vi "FRCts20_Backend_SNS_Subscribe.vi"(6 "Message Attributes":T1, 8 "error in (no error)":errorcluster, 10 "Data":string, 11 "Engine_Refnums":T2) -> (0 "error out":errorcluster)   [LabVIEW 2013, in "FRCts20_Backend_Engine.lvlib"]
uses:
  FRCts20_Backend_Engine.lvlib
  FRCts20_Backend_EngineRefnums.ctl
  INI_Accessor/FRCts20_Backend_INI Controller.lvclass
  Dependencies/AMC/_SubVIs/TypeDefs/Message Queue.ctl
  Dependencies/AMC/_SubVIs/TypeDefs/Message.ctl
  Dependencies/Keyed Array/KeyedArray.ctl
  <vilib>/addons/database/Connection.llb/Conn ObjectReference.ctl
  FRCts20_Backend_FGVOperation.ctl
  FRCts20_Backend_API/FRCts20_Backend_API_SNS.ctl
  <vilib>/National Instruments/NI Amazon Web Services (AWS) Toolkit for LabVIEW/S3/vi source/Typedefs/AMZ_S3_AWS Credentials.ctl
  <vilib>/National Instruments/NI Amazon Web Services (AWS) Toolkit for LabVIEW/SNS/VI Source/AWS SNS Class/AWS_SNS.lvclass
  <vilib>/National Instruments/NI Amazon Web Services (AWS) Toolkit for LabVIEW/SNS/VI Source/Public Typedefs/AWS_SNS Subcribe Parameters.ctl
  <vilib>/National Instruments/NI Amazon Web Services (AWS) Toolkit for LabVIEW/S3/vi source/LV Interface for Amazon S3.lvlib
  <vilib>/National Instruments/NI Amazon Web Services (AWS) Toolkit for LabVIEW/SNS/VI Source/AWS_SNS.lvlib
  FRCts20_Backend_API/FRCts20_Backend_API.lvlib
  Dependencies/Keyed Array/Tools_KeyedArray.lvlib
  Dependencies/AMC/AMC.lvlib
  <vilib>/addons/database/NI_Database_API.lvlib
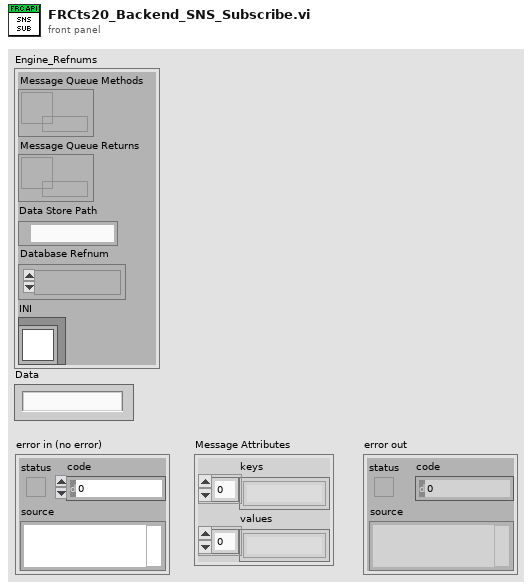
[diagram p1: front panel]
types:
  T1 = typedef "Tools_KeyedArray.lvlib/KeyedArray.ctl" = cluster{"keys":string[], "values":string[]}
  T2 = typedef "FRCts20_Backend_Engine.lvlib/FRCts20_Backend_EngineRefnums.ctl" = cluster{"Message Queue Methods":T3, "Message Queue Returns":T3, "Data Store Path":path, "Database Refnum":T4, "INI":refnum<class "FRCts20_Backend_INI Controller.lvclass">}
  T3 = typedef "AMC.lvlib/Message Queue.ctl" = refnum<queue>
  T4 = typedef "NI_Database_API.lvlib/Conn ObjectReference.ctl" = refnum<k1>
  T5 = typedef "LV Interface for Amazon S3.lvlib/AMZ_S3_AWS Credentials.ctl" = cluster{"Access Key":string, "Secret Key":string}
  T6 = typedef "FRCts20_Backend_API.lvlib/FRCts20_Backend_API_SNS.ctl" = cluster{"Event Name":string, "Team Number":u32, "Subject":string, "Main Message":string, "Phone#":string, "APIReturn":string, "Email":string, "Request Index":u32}
  T7 = typedef "FRCts20_Backend_Engine.lvlib/FRCts20_Backend_FGVOperation.ctl" = enum16{"Initialize", "EnqueueMessage", "EnqueueDataReturn", "FlushMessage", "FlushDataReturn"}
  T8 = typedef "AWS_SNS.lvlib/AWS_SNS Subcribe Parameters.ctl" = cluster{"Endpoint":string, "Protocol":string, "TopicArn":string}
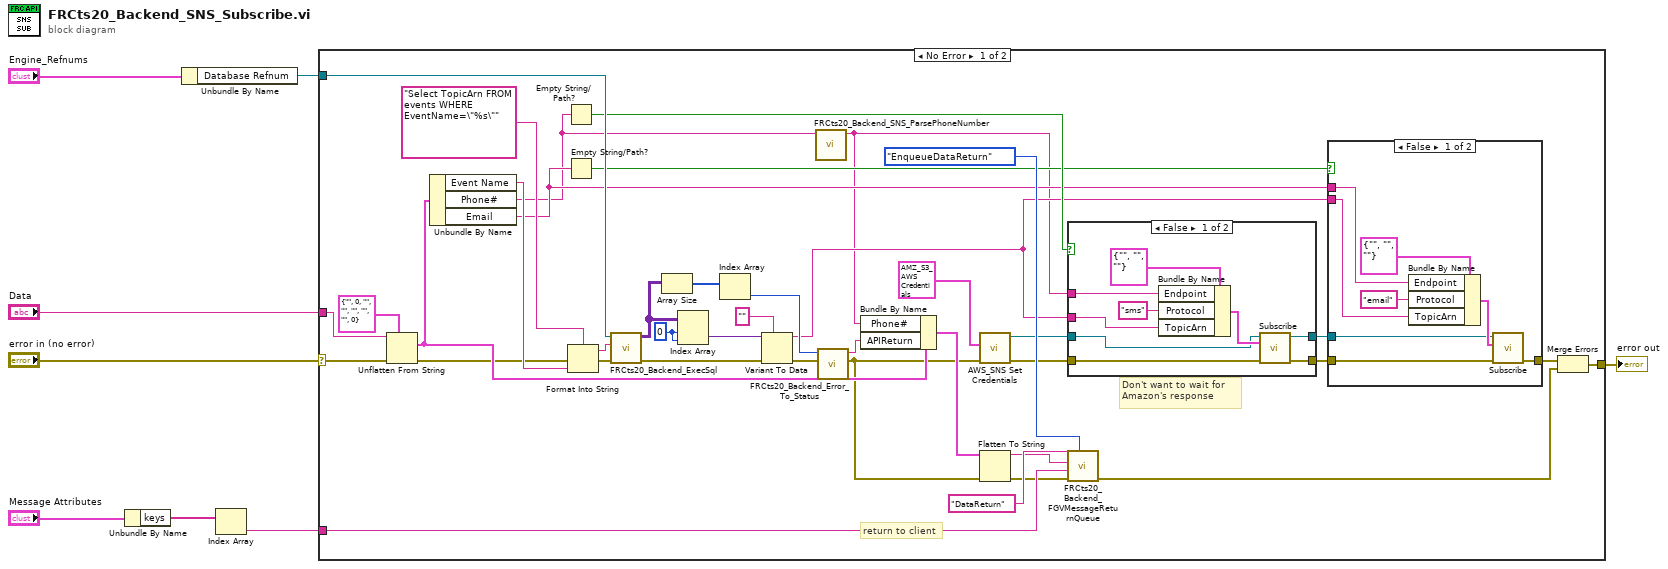
[diagram p0: block diagram]
diagram:
  n1 = Unbundle By Name("Message Attributes") -> ("keys"=w4:string[])
  n2 = Unbundle By Name("Engine_Refnums") -> ("Database Refnum"=w1:T4)
  n3 = Index Array(array=w4) -> (element=w3:string)  [unwired: 1 in]
  n4 = case shown="No Error" "error in (no error)" {
    selector: "error in (no error)" -> [w46 w69]
    tunnel: [w23 w69] -> w7
    tunnel: w1 -> [w35 _]
    tunnel: "Data" -> [w47 _]
    tunnel: w3 -> [w48 _]
    frame No Error {
      w39 = 0 ("index (row)")
      # "Don't want to wait for \nAmazon's response"
      # "return to client"
      n5 = Unflatten From String(type=T6 {"Event Name"="", "Team Number"=0, "Subject"="", "Main Message"="", "Phone#"="", "APIReturn"="", "Email"="", "Request Index"=0} ("SNS"), binary string=w47, error in (no error)=w46) -> (value=w30:T6, error out=w26:errorcluster)  [unwired: 2 in, 1 out]
      n6 = Unbundle By Name(w30) -> ("Event Name"=w34:string, "Phone#"=w10:string, "Email"=w16:string)
      n7 = Empty String/Path?(string/path=w10) -> (empty?=w22:bool)
      n8 = Empty String/Path?(string/path=w16) -> (empty?=w15:bool)
      n9 = Format Into String(format string="Select TopicArn FROM events WHERE EventName=\"%s\"" ("TopicArn"), error in=w26, w34) -> (resulting string=w41:string, error out=w42:errorcluster)  [unwired: 1 in]
      n10 = call "FRCts20_Backend_ExecSql.vi"("error in (no error)"=w42, "format string"=w41, "Refnum in"=w35) -> ("error out"=w43:errorcluster, "recordset data"=w33:variant[][])  [unwired: 6 in, 1 out]
      n11 = Array Size(array=w33) -> (size(s)=w32:i32[])
      n12 = Index Array(array=w33, index (row)=w39, index (col)=w39) -> (element=w38:variant)
      n13 = Index Array(array=w32) -> (element=w31:i32)  [unwired: 1 in]
      n14 = Variant To Data(error in=w43, type="" ("TopicArn"), Variant=w38) -> (data=w17:string, error out=w12:errorcluster)
      n15 = call "FRCts20_Backend_SNS_ParsePhoneNumber.vi"("Phone# In"=w10) -> ("Phone# Out"=w9:string)  [unwired: 10 in]
      n16 = call "FRCts20_Backend_Error_To_Status.vi"("error in (no error)"=w12, "rows affected"=w31) -> ("error out"=w11:errorcluster, "String"=w29:string)  [unwired: 8 in]
      n17 = Bundle By Name(cluster=w30, "Phone#"=w9, "APIReturn"=w29) -> (w28:T6)
      n18 = call <vilib>:"AWS_SNS Set Credentials.vi"("error in (no error)"=w11, "AWS Credentials"=T5 {"Access Key"="AKIAIBWID7GQA3ZVLBGQ", "Secret Key"="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"} ("AWS Credentials in")) -> ("error out"=w20:errorcluster, "AWS_SNS.lvlib:AWS_SNS.lvclass"=w19:refnum<class "AWS_SNS.lvclass">)  [unwired: 8 in]
      n19 = Flatten To String(anything=w28, error in (no error)=w11) -> (data string=w27:string, error out=w25:errorcluster)  [unwired: 2 in, 1 out]
      n20 = case shown="False" w22 {
        tunnel: w17 -> [w63 _]
        tunnel: w9 -> [w62 _]
        tunnel: [w61 w68] -> w18
        tunnel: [w60 w67] -> w14
        tunnel: w20 -> [w59 w68]
        tunnel: w19 -> [w58 w67]
        frame False {
          n21 = Bundle By Name(cluster=T8 {"Endpoint"="", "Protocol"="", "TopicArn"=""} ("Subscribe Parameters"), "Endpoint"=w62, "Protocol"="sms", "TopicArn"=w63) -> (w66:T8)
          n22 = call-dynamic "Subscribe.vi"("error in (no error)"=w59, "Subscribe Parameters"=w66, "AWS_SNS.lvlib:AWS_SNS.lvclass"=w58) -> ("error out"=w61:errorcluster, "AWS_SNS.lvlib:AWS_SNS.lvclass"=w60:refnum<class "AWS_SNS.lvclass">)  [unwired: 6 in, 1 out]
        }
        frame True {
        }
      }
      n23 = call "FRCts20_Backend_FGVMessageReturnQueue.vi"("Operation"=FRCts20_Backend_FGVOperation."EnqueueDataReturn", "error in (no error)"=w25, "Key"=w48, "Message Value"=w27, "Message Name"="DataReturn") -> ("error out"=w24:errorcluster)  [unwired: 5 in, 1 out]
      n24 = case shown="False" w15 {
        tunnel: w17 -> [w53 _]
        tunnel: w16 -> [w52 _]
        tunnel: [w51 w57] -> w13
        tunnel: w18 -> [w50 w57]
        tunnel: w14 -> [w49 _]
        frame False {
          n25 = Bundle By Name(cluster=T8 {"Endpoint"="", "Protocol"="", "TopicArn"=""} ("Subscribe Parameters"), "Endpoint"=w52, "Protocol"="email", "TopicArn"=w53) -> (w56:T8)
          n26 = call-dynamic "Subscribe.vi"("error in (no error)"=w50, "Subscribe Parameters"=w56, "AWS_SNS.lvlib:AWS_SNS.lvclass"=w49) -> ("error out"=w51:errorcluster)  [unwired: 6 in, 2 out]
        }
        frame True {
        }
      }
      n27 = Merge Errors(w13, w24) -> (w23:errorcluster)
    }
    frame Error {
    }
  }
  "error out" <- w7
